vi "Status Position.vi"(0 "status":i32, 1 "error in (no error)":errorcluster) -> (2 "status out":i32, 3 "function return":i32, 4 "error out":errorcluster)   [LabVIEW 2014, in "MCM3000.lvlib"]
doc: "long StatusPosition(long &status);"
uses:
  MCM3000.lvlib
  ThorMCM3000.dll
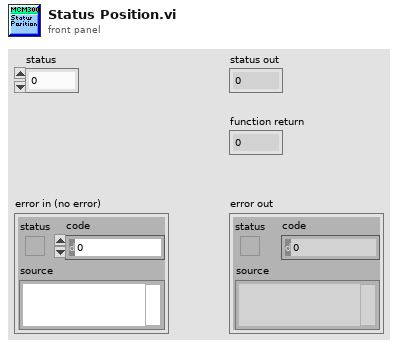
[diagram p1: front panel]
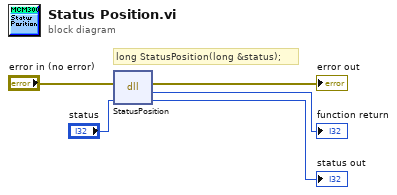
[diagram p0: block diagram]
diagram:
  # "long StatusPosition(long &status);"
  n1 = dll-call lib="C:/TIS_CalebVS2012/TIS_Development/Hardware/SDKs/MCM3000_SDK/LabVIEW/inc/ThorMCM3000.*" fn="StatusPosition"(error in="error in (no error)", "status"="status") -> (error out=→"error out":errorcluster, →"function return":i32, "status"=→"status out":i32)  [unwired: 2 in, 1 out]
